vi "WiiMote Pair.vi"(8 "error in (no error)":errorcluster) -> (0 "error out":errorcluster, 2 "Log":string[](array[string]))   [LabVIEW 2012]
doc: "Pairs a WiiMote by MAC address."
uses:
  C:/WINNT/system32/InTheHand.Net.Personal.dll
  WINNT/system32/InTheHand.Net.Personal.dll
panel:
  in  "MAC address to pair":string
  in  "Bluetooth Security 2":refnum<k24>
  out "Client":refnum<k24>
  in  "System.Timespan":refnum<k24>
  in  "Log":i32(listbox)=1
  in  "Bluetooth Security":refnum<k24>
  in  "Bluetooth Service":refnum<k24>
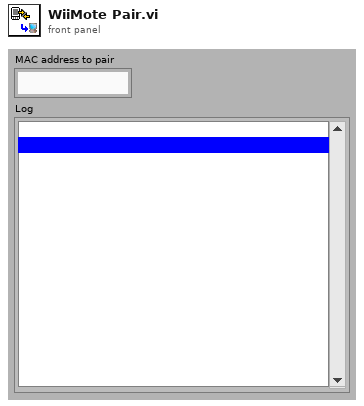
[diagram p1: front panel]
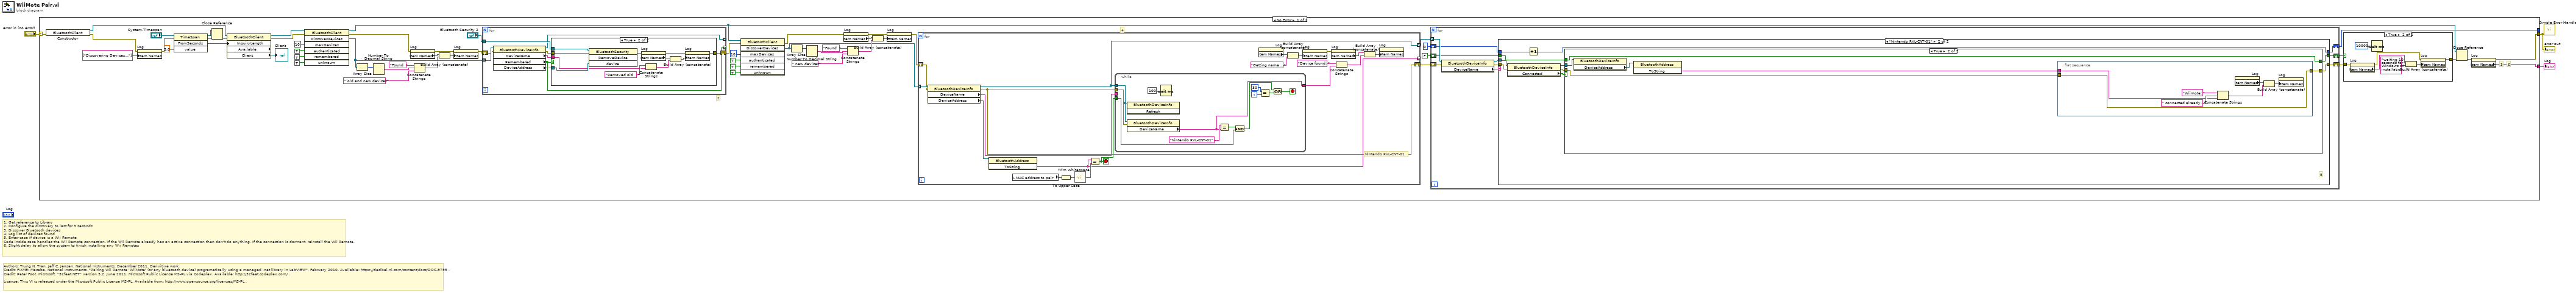
[diagram p0: block diagram]
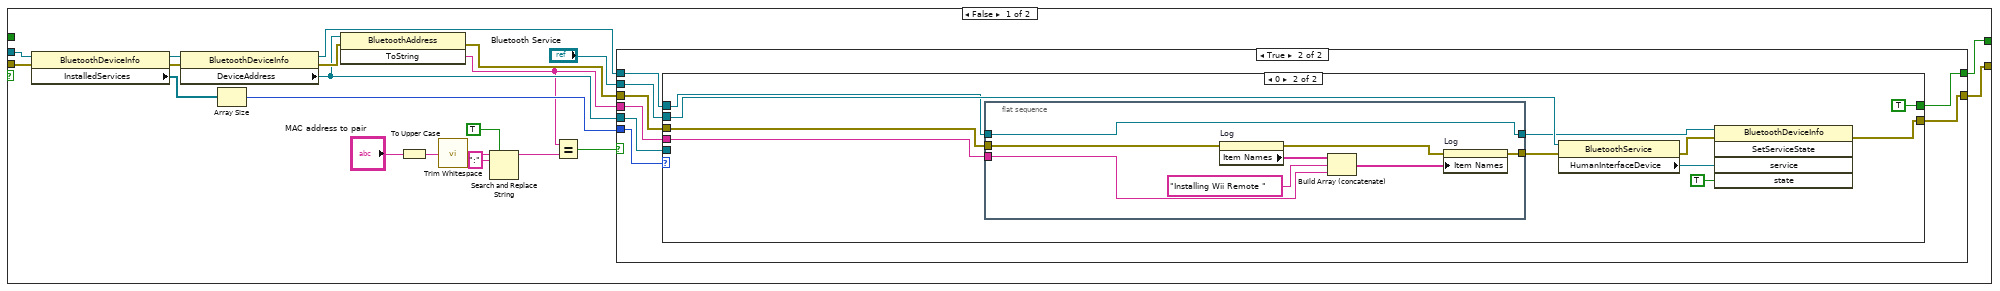
[diagram p5: hidden frame]
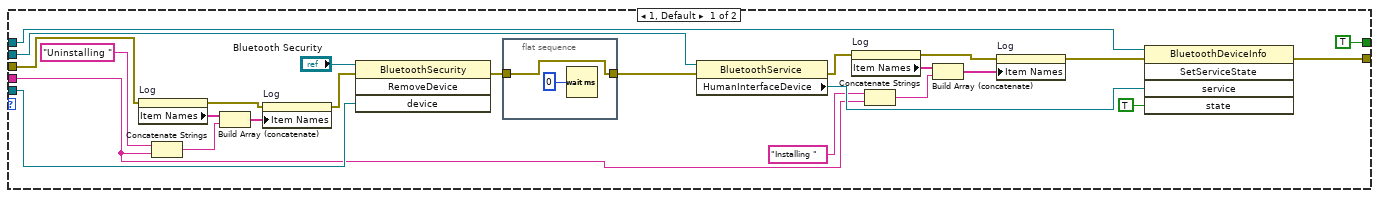
[diagram p7: hidden frame]
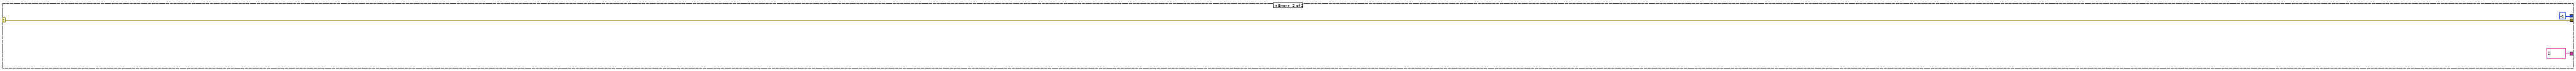
[diagram p8: hidden frame]
diagram:
  # "Authors: Trung N. Tran, Jeff C. Jensen, National Instruments, December 2011. Derivitive work.\nCredit: FIXME: Macaba, National Instruments, \"Pairing Wii Remote 'WiiMote' (or any bluetooth device) programatically using a managed .net library in LabVIEW\", February 2010. Available: https://decibel.ni.com/content/docs/DOC-9799 .\nCredit: Peter Foot, Microsoft, \"32feet.NET\" version 3.2, June 2011. Microsoft Public License MS-PL via Codeplex. Available: http://32feet.codeplex.com/ .\n\nLicense: This VI is released under the Microsoft Public License MS-PL. Available from: http://www.opensource.org/licenses/MS-PL ."
  # "1. Get reference to Library\n2. Configure the discovery to last for 3 seconds\n3. Discover Bluetooth devices\n4. Log list of devices found\n5. Enter case if device is a Wii Remote\nCode inside case handles the Wii Remote connection. If the Wii Remote already has an active connection then don't do anything. If the connection is dormant, reinstall the Wii Remote.\n6. Slight delay to allow the system to finish installing any Wii Remotes"
  n1 = case shown="No Error" "error in (no error)" {
    selector: "error in (no error)" -> [w50 w237]
    tunnel: [w52 w237] -> w1
    tunnel: [w51 string[] [] ("Item Names")] -> w3
    tunnel: [w49 -1] -> _
    frame No Error {
      # "6"
      # "4"
      # "3"
      # "2"
      n2 = constructor class="BluetoothClient"(error in=w50) -> (reference out=w48:refnum<k24>, error out=w55:errorcluster)  [unwired: 2 in, 1 out]
      n3 = property on="Log" class="LstBox (strict)"(error in=w55, "Item Names"=string[] ["Discovering Devices..."]) -> (error out=w39:errorcluster)  [unwired: 1 in, 1 out]
      n4 = invoke class="TimeSpan" method="FromSeconds"(reference="System.Timespan", error in=w39, "value"=3.0) -> (reference out=w43:refnum<k24>, error out=w42:errorcluster, "FromSeconds"=w44:refnum<k24>)  [unwired: 1 in, 1 out]
      n5 = Close Reference(reference=w43, error in (no error)=w42) -> (error out=w41:errorcluster)
      n6 = property class="BluetoothClient" props=["InquiryLength", "Available", "Client"](reference=w48, error in=w41, "InquiryLength"=w44) -> (reference out=w47:refnum<k24>, error out=w40:errorcluster, "Client"=→"Client":refnum<k24>)  [unwired: 1 out]
      n7 = invoke class="BluetoothClient" method="DiscoverDevices"(reference=w47, error in=w40, "maxDevices"=10, "authenticated"=TRUE, "remembered"=TRUE, "unknown"=TRUE) -> (reference out=w7:refnum<k24>, error out=w13:errorcluster, "DiscoverDevices"=w15:refnum<k24>[])  [unwired: 1 in, 4 out]
      n8 = Array Size(array=w15) -> (size(s)=w16:i32)
      n9 = Number To Decimal String(number=w16) -> (decimal integer string=w18:string)  [unwired: 1 in]
      n10 = property on="Log" class="LstBox (strict)"(error in=w13) -> (error out=w20:errorcluster, "Item Names"=w22:string[])  [unwired: 1 in, 1 out]
      n11 = Concatenate Strings("Found  ", w18, " old and new devices" ("element")) -> (w14:string)
      n12 = Build Array (concatenate)(w22, w14) -> (w21:string[])
      n13 = property on="Log" class="LstBox (strict)"(error in=w20, "Item Names"=w21) -> (error out=w12:errorcluster)  [unwired: 1 in, 1 out]
      n14 = for {
        tunnel: w15 -> [w70] mode=indexing
        tunnel: [w68] -> _ mode=indexing
        tunnel: "Bluetooth Security 2" -> [w69]
        tunnel: [w66] -> _ mode=indexing
        shift-right: [w62] -> w5
        shift-left: w12 -> [w65]
        n15 = property class="BluetoothDeviceInfo"(reference=w70, error in=w65) -> (reference out=w66:refnum<k24>, error out=w64:errorcluster, "DeviceName"=w63:string, "Remembered"=w68:bool, "DeviceAddress"=w67:refnum<k24>)
        n16 = case shown="True" w68 {
          tunnel: w69 -> [_ w82]
          tunnel: w67 -> [_ w81]
          tunnel: w64 -> [w71 w74]
          tunnel: w63 -> [_ w76]
          tunnel: [w71 w72] -> w62
          frame False {
          }
          frame True {
            n17 = invoke class="BluetoothSecurity" method="RemoveDevice"(reference=w82, error in=w74, "device"=w81) -> (error out=w73:errorcluster)  [unwired: 1 in, 3 out]
            n18 = property on="Log" class="LstBox (strict)"(error in=w73) -> (error out=w80:errorcluster, "Item Names"=w78:string[])  [unwired: 1 in, 1 out]
            n19 = Concatenate Strings("Removed old    ", w76) -> (w75:string)
            n20 = Build Array (concatenate)(w78, w75) -> (w79:string[])
            n21 = property on="Log" class="LstBox (strict)"(error in=w80, "Item Names"=w79) -> (error out=w72:errorcluster)  [unwired: 1 in, 1 out]
          }
        }
      }
      n22 = invoke class="BluetoothClient" method="DiscoverDevices"(reference=w7, error in=w5, "maxDevices"=10, "authenticated"=TRUE, "remembered"=TRUE, "unknown"=TRUE) -> (error out=w4:errorcluster, "DiscoverDevices"=w6:refnum<k24>[])  [unwired: 1 in, 5 out]
      n23 = Array Size(array=w6) -> (size(s)=w34:i32)
      n24 = Number To Decimal String(number=w34) -> (decimal integer string=w32:string)  [unwired: 1 in]
      n25 = property on="Log" class="LstBox (strict)"(error in=w4) -> (error out=w35:errorcluster, "Item Names"=w37:string[])  [unwired: 1 in, 1 out]
      n26 = Concatenate Strings("Found  ", w32, " new devices" ("element")) -> (w30:string)
      n27 = Build Array (concatenate)(w37, w30) -> (w36:string[])
      n28 = property on="Log" class="LstBox (strict)"(error in=w35, "Item Names"=w36) -> (error out=w23:errorcluster)  [unwired: 1 in, 1 out]
      n29 = for {
        tunnel: w6 -> [w102] mode=indexing
        tunnel: [w94] -> w38 mode=indexing
        shift-right: [w95] -> w57
        shift-left: w23 -> [w101]
        tunnel: [w85] -> _ mode=indexing
        stop <- w83 stop-if-true
        # "Nintendo RVL-CNT-01"
        n30 = property class="BluetoothDeviceInfo"(reference=w102, error in=w101) -> (reference out=w94:refnum<k24>, error out=w95:errorcluster, "DeviceName"=w89:string, "DeviceAddress"=w88:refnum<k24>)
        n31 = invoke class="BluetoothAddress" method="ToString"(reference=w88) -> ("ToString"=w85:string)  [unwired: 2 in, 2 out]
        n32 = local read "MAC address to pair"() -> (w84:string)
        n33 = To Upper Case(1:w84) -> (0:w87:string)
        n34 = call <vilib>:"Trim Whitespace.vi"("string"=w87) -> ("trimmed string"=w86:string)  [unwired: 1 in]
        n35 = Equal?(x=w85, y=w86) -> (x = y?=w83:bool)
        n36 = while {
          tunnel: w89 -> [_]
          tunnel: [w108] -> w96
          tunnel: w95 -> [w114]
          tunnel: w94 -> [w113]
          tunnel: w83 -> [w106]
          i -> [w110]
          stop <- w103 stop-if-true
          n37 = invoke class="BluetoothDeviceInfo" method="Refresh"(reference=w113) -> ()  [unwired: 2 in, 3 out]
          n38 = property class="BluetoothDeviceInfo"(reference=w113, error in=w114) -> ("DeviceName"=w108:string)  [unwired: 2 out]
          n39 = Wait (ms)(milliseconds to wait=u32 100) -> ()  [unwired: 1 out]
          n40 = Equal?(x="Nintendo RVL-CNT-01" ("ToString"), y=w108) -> (x = y?=w107:bool)
          n41 = And(x=w107, y=w106) -> (x .and. y?=w105:bool)
          n42 = Equal?(x=30, y=w110) -> (x = y?=w104:bool)
          n43 = Or(x=w105, y=w104) -> (x .or. y?=w103:bool)
        }
        n44 = property on="Log" class="LstBox (strict)"() -> ("Item Names"=w92:string[])  [unwired: 2 in, 2 out]
        n45 = Build Array (concatenate)(w92, "Getting name ...") -> (w93:string[])
        n46 = property on="Log" class="LstBox (strict)"("Item Names"=w93) -> (error out=w91:errorcluster)  [unwired: 2 in, 1 out]
        n47 = property on="Log" class="LstBox (strict)"(error in=w91) -> ("Item Names"=w100:string[])  [unwired: 1 in, 2 out]
        n48 = Concatenate Strings("Device found: ", w96) -> (w98:string)
        n49 = Build Array (concatenate)(w100, w98) -> (w99:string[])
        n50 = property on="Log" class="LstBox (strict)"("Item Names"=w99) -> ()  [unwired: 2 in, 2 out]
      }
      n51 = for {
        shift-right: [w129] -> w58
        shift-left: w57 -> [w130]
        tunnel: w38 -> [w127] mode=indexing
        shift-right: [w126] -> w60
        shift-left: FALSE -> [w125]
        shift-right: [w123] -> w49
        shift-left: 0 -> [w124]
        n52 = property class="BluetoothDeviceInfo"(reference=w127, error in=w130) -> (reference out=w131:refnum<k24>, error out=w128:errorcluster, "DeviceName"=w132:string)
        n53 = case shown="\"Nintendo RVL-CNT-01\"" w132 {
          tunnel: w131 -> [_ w145]
          tunnel: [w135 w142] -> w129
          tunnel: w128 -> [w135 w141]
          tunnel: [w134 w139] -> w126
          tunnel: w125 -> [w134 w138]
          tunnel: w124 -> [w133 w137]
          tunnel: [w133 w136] -> w123
          frame "", Default {
          }
          frame "Nintendo RVL-CNT-01" {
            # "5"
            n54 = property class="BluetoothDeviceInfo"(reference=w145, error in=w141) -> (reference out=w143:refnum<k24>, error out=w140:errorcluster, "Connected"=w144:bool)
            n55 = Increment(x=w137) -> (x+1=w136:i32)
            n56 = case shown="True" w144 {
              tunnel: w143 -> [w166 w225]
              tunnel: [w162 w226] -> w142
              tunnel: w140 -> [w161 w227]
              tunnel: [w160 w222] -> w139
              tunnel: w138 -> [_ w222]
              frame False {
                n57 = property class="BluetoothDeviceInfo"(reference=w166, error in=w161) -> (reference out=w155:refnum<k24>, error out=w154:errorcluster, "InstalledServices"=w165:refnum<k24>[])
                n58 = property class="BluetoothDeviceInfo"(reference=w155, error in=w154) -> (reference out=w156:refnum<k24>, error out=w159:errorcluster, "DeviceAddress"=w158:refnum<k24>)
                n59 = Array Size(array=w165) -> (size(s)=w164:i32)
                n60 = invoke class="BluetoothAddress" method="ToString"(reference=w158, error in=w159) -> (error out=w157:errorcluster, "ToString"=w153:string)  [unwired: 1 in, 1 out]
                n61 = To Upper Case(1:"MAC address to pair") -> (0:w150:string)
                n62 = call <vilib>:"Trim Whitespace.vi"("string"=w150) -> ("trimmed string"=w149:string)  [unwired: 1 in]
                n63 = Search and Replace String(replace all?=TRUE ("replace all? (F)"), input string=w149, search string=":") -> (result string=w146:string)  [unwired: 5 in, 3 out]
                n64 = Equal?(x=w153, y=w146) -> (x = y?=w151:bool)
                n65 = case shown="True" w151 {
                  tunnel: w164 -> [_ w175]
                  tunnel: "Bluetooth Service" -> [_ w174]
                  tunnel: [w167 w173] -> w162
                  tunnel: [_ w172] -> w160
                  tunnel: w158 -> [_ w171]
                  tunnel: w157 -> [w167 w170]
                  tunnel: w156 -> [_ w169]
                  tunnel: w153 -> [_ w168]
                  frame False {
                  }
                  frame True {
                    n66 = case shown="0" w175 {
                      tunnel: w174 -> [w197 w211]
                      tunnel: [w180 w209] -> w173
                      tunnel: w170 -> [w177 w207]
                      tunnel: [TRUE ("state") TRUE ("state")] -> w172
                      tunnel: w171 -> [w179 _]
                      tunnel: w169 -> [w178 w204]
                      tunnel: w168 -> [w176 w203]
                      frame 1, Default {
                        n67 = property on="Log" class="LstBox (strict)"(error in=w177) -> (error out=w190:errorcluster, "Item Names"=w192:string[])  [unwired: 1 in, 1 out]
                        n68 = Concatenate Strings("Uninstalling ", w176) -> (w187:string)
                        n69 = Build Array (concatenate)(w192, w187) -> (w191:string[])
                        n70 = property on="Log" class="LstBox (strict)"(error in=w190, "Item Names"=w191) -> (error out=w184:errorcluster)  [unwired: 1 in, 1 out]
                        n71 = invoke class="BluetoothSecurity" method="RemoveDevice"(reference="Bluetooth Security", error in=w184, "device"=w179) -> (error out=w183:errorcluster)  [unwired: 1 in, 3 out]
                        n72 = flat-sequence {
                          tunnel: w183 -> [w201]
                          tunnel: [w201] -> w189
                          frame #0 {
                            n73 = Wait (ms)(milliseconds to wait=u32 0) -> ()  [unwired: 1 out]
                          }
                        }
                        n74 = property class="BluetoothService"(reference=w197, error in=w189) -> (error out=w182:errorcluster, "HumanInterfaceDevice"=w198:refnum<k24>)  [unwired: 1 out]
                        n75 = property on="Log" class="LstBox (strict)"(error in=w182) -> (error out=w193:errorcluster, "Item Names"=w194:string[])  [unwired: 1 in, 1 out]
                        n76 = Concatenate Strings("Installing ", w176) -> (w185:string)
                        n77 = Build Array (concatenate)(w194, w185) -> (w195:string[])
                        n78 = property on="Log" class="LstBox (strict)"(error in=w193, "Item Names"=w195) -> (error out=w181:errorcluster)  [unwired: 1 in, 1 out]
                        n79 = invoke class="BluetoothDeviceInfo" method="SetServiceState"(reference=w178, error in=w181, "service"=w198, "state"=TRUE) -> (error out=w180:errorcluster)  [unwired: 1 in, 4 out]
                      }
                      frame 0 {
                        n80 = flat-sequence {
                          tunnel: [w214] -> w208
                          tunnel: w207 -> [w216]
                          tunnel: [w218] -> w205
                          tunnel: w204 -> [w218]
                          tunnel: w203 -> [w217]
                          frame #0 {
                            n81 = property on="Log" class="LstBox (strict)"(error in=w216) -> (error out=w215:errorcluster, "Item Names"=w220:string[])  [unwired: 1 in, 1 out]
                            n82 = Build Array (concatenate)(w220, "Installing Wii Remote " ("Status"), w217) -> (w219:string[])
                            n83 = property on="Log" class="LstBox (strict)"(error in=w215, "Item Names"=w219) -> (error out=w214:errorcluster)  [unwired: 1 in, 1 out]
                          }
                        }
                        n84 = property class="BluetoothService"(reference=w211, error in=w208) -> (error out=w210:errorcluster, "HumanInterfaceDevice"=w212:refnum<k24>)  [unwired: 1 out]
                        n85 = invoke class="BluetoothDeviceInfo" method="SetServiceState"(reference=w205, error in=w210, "service"=w212, "state"=TRUE) -> (error out=w209:errorcluster)  [unwired: 1 in, 4 out]
                      }
                    }
                  }
                }
              }
              frame True {
                n86 = property class="BluetoothDeviceInfo"(reference=w225) -> ("DeviceAddress"=w224:refnum<k24>)  [unwired: 1 in, 2 out]
                n87 = invoke class="BluetoothAddress" method="ToString"(reference=w224) -> ("ToString"=w223:string)  [unwired: 2 in, 2 out]
                n88 = flat-sequence {
                  tunnel: [w234] -> w226
                  tunnel: w227 -> [w234]
                  tunnel: w223 -> [w233]
                  frame #0 {
                    n89 = Concatenate Strings("Wiimote: " ("string"), w233, " connected already..." ("string")) -> (w230:string)
                    n90 = property on="Log" class="LstBox (strict)"() -> ("Item Names"=w229:string[])  [unwired: 2 in, 2 out]
                    n91 = Build Array (concatenate)(w229, w230) -> (w228:string[])
                    n92 = property on="Log" class="LstBox (strict)"("Item Names"=w228) -> ()  [unwired: 2 in, 2 out]
                  }
                }
              }
            }
          }
        }
      }
      n93 = case shown="True" w60 {
        tunnel: [w115 w118] -> w59
        tunnel: w58 -> [w115 w117]
        frame False {
        }
        frame True {
          n94 = property on="Log" class="LstBox (strict)"(error in=w117) -> (error out=w116:errorcluster, "Item Names"=w121:string[])  [unwired: 1 in, 1 out]
          n95 = Wait (ms)(milliseconds to wait=u32 10000) -> ()  [unwired: 1 out]
          n96 = Build Array (concatenate)(w121, "waiting 10 seconds for Windows driver installation..." ("Status")) -> (w119:string[])
          n97 = property on="Log" class="LstBox (strict)"(error in=w116, "Item Names"=w119) -> (error out=w118:errorcluster)  [unwired: 1 in, 1 out]
        }
      }
      n98 = Close Reference(reference=w7, error in (no error)=w59) -> (error out=w53:errorcluster)
      n99 = property on="Log" class="LstBox (strict)"(error in=w53) -> (error out=w52:errorcluster, "Item Names"=w51:string[])  [unwired: 1 in, 1 out]
    }
    frame Error {
    }
  }
  "error out" <- w1
  "Log" <- w3
  n100 = call <vilib>:"Simple Error Handler.vi"("error in (no error)"=w1) -> ()  [unwired: 4 in, 5 out]
